vi "Get Just Validate.vi"(8 "error in (no error)":errorcluster, 11 "CFG JSON Base in":refnum<class "CFG JSON Base.lvclass">) -> (0 "error out":errorcluster, 2 "Just Validate":bool, 3 "CFG JSON Base out":refnum<class "CFG JSON Base.lvclass">)   [LabVIEW 2023, in "HAL GOOP4.lvlib" / "CFG JSON Base.lvclass"]
uses:
  CFG JSON Base.lvclass
  CFG JSON Base.lvclass/CFG JSON Base.ctl
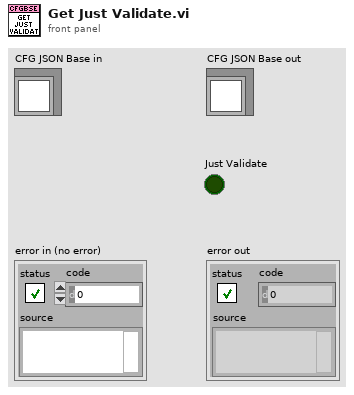
[diagram p1: front panel]
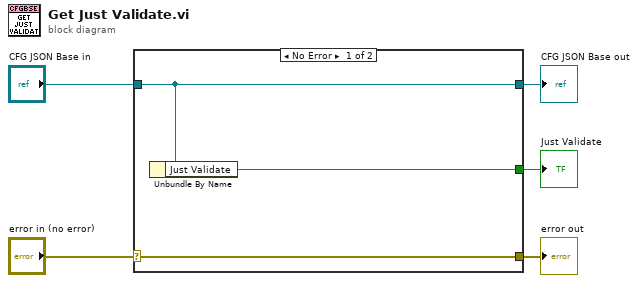
[diagram p0: block diagram]
diagram:
  n1 = case shown="No Error" "error in (no error)" {
    selector: "error in (no error)" -> [w8 w9]
    tunnel: [w8 w9] -> w4
    tunnel: [w7 w10] -> w2
    tunnel: "CFG JSON Base in" -> [w7 w10]
    tunnel: [w6 _] -> w1
    frame No Error {
      n2 = Unbundle By Name(w7) -> ("Just Validate"=w6:bool)
    }
    frame Error {
    }
  }
  "error out" <- w4
  "CFG JSON Base out" <- w2
  "Just Validate" <- w1
